vi "set_delay_chirp_TRIG1.vi"(5 "background period":dbl=5e-06, 7 "molecular delay":dbl min=0.0 max=999.999999999995 format="%.12f", 8 "error in":errorcluster, 11 "VISA resource name":refnum<visa-resource-name>) -> (0 "error out":errorcluster, 3 "VISA resource name out":refnum<visa-resource-name>)   [LabVIEW 2011]
doc: "This subVI sets the delay of the output channels relative to other channels or to the time reference T0 .\nControls A=, B= , C= and D= specify the reference channel and \nA, B, C, and D set the delay time in seconds .\nA Delay Linkage Error will be caused by an attempt to totally disconnect a time reference from T0 ."
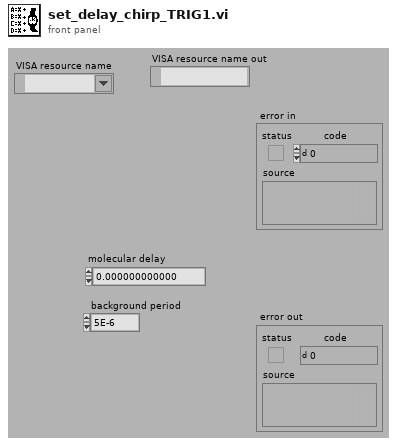
[diagram p1: front panel]
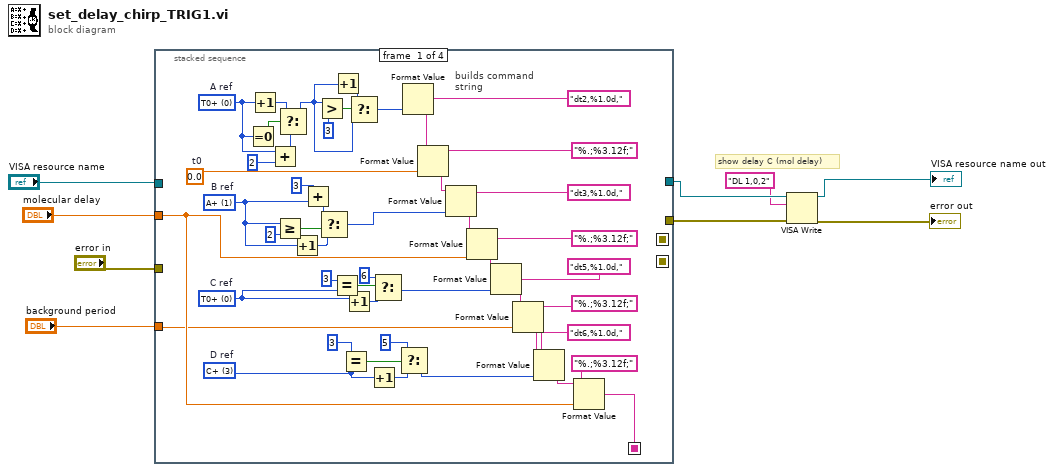
[diagram p0: block diagram]
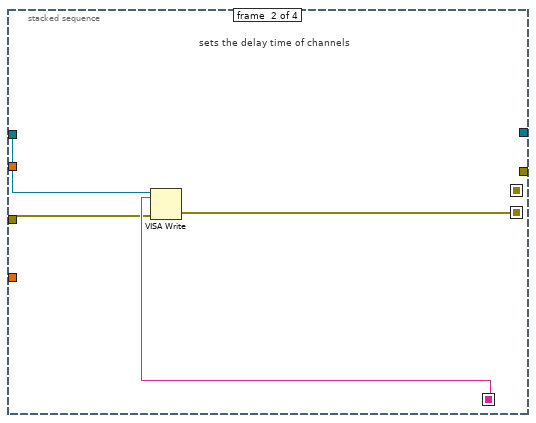
[diagram p2: hidden frame]
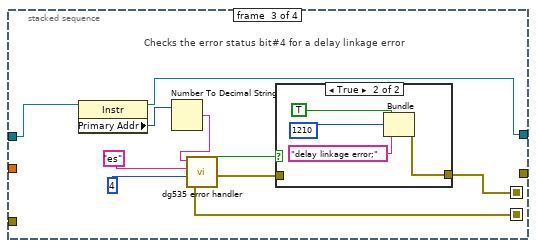
[diagram p3: hidden frame]
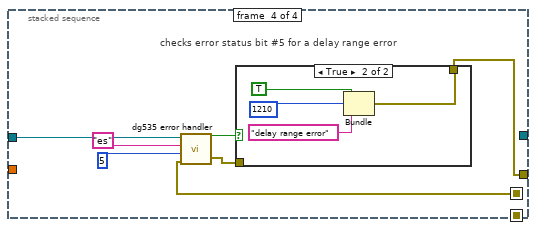
[diagram p5: hidden frame]
diagram:
  # "show delay C (mol delay)"
  n1 = stacked-sequence {
    seq-local: [w42 _ _ _] -> [_ w61 _ _]
    seq-local: [_ w59 _ _] -> [_ _ w71 _]
    seq-local: [_ _ w68 _] -> [_ _ _ w77]
    tunnel: "VISA resource name" -> [_ w58 w65 w80]
    tunnel: "error in" -> [_ w60 _ _]
    tunnel: [_ _ _ w81] -> w7
    tunnel: [_ _ w62 _] -> w5
    tunnel: "molecular delay" -> [w11 _ _ _]
    tunnel: "background period" -> [w10 _ _ _]
    frame #0 {
      w55 = 0.0  # t0
      w37 = u32 3 items=["T0+", "A+", "B+", "C+"]  # D ref
      w31 = u32 0 items=["T0+", "A+", "B+", "D+"]  # C ref
      w12 = u32 1 items=["T0+", "A+", "C+", "D+"]  # B ref
      w22 = u32 0 items=["T0+", "B+", "C+", "D+"]  # A ref
      # "builds command\nstring"
      n2 = Equal To 0?(x=w22) -> (x = 0?=w23:bool)
      n3 = Increment(x=w22) -> (x+1=w14:u32)
      n4 = Add(x=w22, y=2) -> (x+y=w20:u32)
      n5 = Greater Or Equal?(x=w12, y=2) -> (x >= y?=w26:bool)
      n6 = Select(t=w14, s=w23, f=w20) -> (s? t:f=w13:u32)
      n7 = Increment(x=w12) -> (x+1=w24:u32)
      n8 = Add(x=3, y=w12) -> (x+y=w27:u32)
      n9 = Greater?(x=w13, y=3) -> (0:w18:bool)
      n10 = Select(t=w27, s=w26, f=w24) -> (s? t:f=w25:u32)
      n11 = Equal?(x=3, y=w31) -> (x = y?=w34:bool)
      n12 = Increment(x=w13) -> (x+1=w17:u32)
      n13 = Equal?(x=3, y=w37) -> (x = y?=w39:bool)
      n14 = Increment(x=w31) -> (x+1=w30:u32)
      n15 = Select(t=w17, s=w18, f=w13) -> (s? t:f=w16:u32)
      n16 = Increment(x=w37) -> (x+1=w32:u32)
      n17 = Select(t=6, s=w34, f=w30) -> (s? t:f=w29:u32)
      n18 = Select(t=5, s=w39, f=w32) -> (s? t:f=w36:u32)
      n19 = Format Value(format string="dt2,%1.0d,", value (0)=w16) -> (output string=w51:string)  [unwired: 1 in]
      n20 = Format Value(string ("")=w51, format string="%.;%3.12f;", value (0)=w55) -> (output string=w50:string)
      n21 = Format Value(string ("")=w50, format string="dt3,%1.0d,", value (0)=w25) -> (output string=w53:string)
      n22 = Format Value(string ("")=w53, format string="%.;%3.12f;", value (0)=w11) -> (output string=w41:string)
      n23 = Format Value(string ("")=w41, format string="dt5,%1.0d,", value (0)=w29) -> (output string=w45:string)
      n24 = Format Value(string ("")=w45, format string="%.;%3.12f;", value (0)=w10) -> (output string=w43:string)
      n25 = Format Value(string ("")=w43, format string="dt6,%1.0d,", value (0)=w36) -> (output string=w48:string)
      n26 = Format Value(string ("")=w48, format string="%.;%3.12f;", value (0)=w11) -> (output string=w42:string)
    }
    frame #1 {
      # "sets the delay time of channels"
      n27 = VISA Write(VISA resource name=w58, write buffer=w61, error in (no error)=w60) -> (error out=w59:errorcluster)  [unwired: 2 out]
    }
    frame #2 {
      # "Checks the error status bit#4 for a delay linkage error"
      n28 = property class="Instr"(reference=w65) -> (reference out=w62:refnum<visa-resource-name>, "Primary Addr"=w64:u16)  [unwired: 1 in, 1 out]
      n29 = Number To Decimal String(number=w64) -> (decimal integer string=w63:string)  [unwired: 1 in]
      n30 = call "dg535 error handler.vi"("error in"=w71, "check bit #"=4, "command string"="es", "GPIB address"=w63) -> ("error out"=w69:errorcluster, "error found"=w70:bool)
      n31 = case shown="True" w70 {
        tunnel: w69 -> [w72 _]
        tunnel: [w72 w73] -> w68
        frame False {
        }
        frame True {
          n32 = Bundle(TRUE, 1210, "delay linkage error;") -> (w73:errorcluster)  [unwired: 1 in]
        }
      }
    }
    frame #3 {
      # "checks error status bit #5 for a delay range error"
      n33 = call "dg535 error handler.vi"("error in"=w77, "check bit #"=5, "command string"="es", "GPIB address"=w80) -> ("error out"=w82:errorcluster, "error found"=w83:bool)
      n34 = case shown="True" w83 {
        tunnel: w82 -> [w84 _]
        tunnel: [w84 w85] -> w81
        frame False {
        }
        frame True {
          n35 = Bundle(TRUE, 1210, "delay range error") -> (w85:errorcluster)  [unwired: 1 in]
        }
      }
    }
  }
  n36 = VISA Write(VISA resource name=w5, write buffer="DL 1,0,2", error in (no error)=w7) -> (VISA resource name out=→"VISA resource name out":refnum<visa-resource-name>, error out=→"error out":errorcluster)  [unwired: 1 out]
